vi "Umrechnung_Koordinaten.vi"(7 "Anderer Winkel":sgl, 8 "error in":errorcluster, 9 "Richtung":enum16{"Kamera nach Real", "Real nach Kamera"}(ring), 10 "Koordinaten in":cluster{"X":sgl, "Y":sgl}, 11 "Cluster in":T1={"Initialisierung"={"Online?"=FALSE, "Grundpfad"=path "", "Kamera Oben"="", "IP-Adresse Flüssiglinse"="", "Flüssiglinse"=refnum, "Kamera Unten"="", "IP-Adresse SPS"="", "SPS-Verbindung"={"TCP Connection Ref"=refnum, "IP address"="", "timeout ms"=5000, "Connected?"=FALSE, "PLC Type"=enum."S7 1200", "Rack S7 400"=0, "Slot S7 400"=0, "PDU Size"=0, "connection semaphore"=refnum}, "IP-Adresse Lichtgitter"="", "Lichtgitter"=refnum, "Skalierungsfaktor"=0.0, "Bilder Oben"=[], "Bild Unten"=refnum, "Bild Ausschnitt Unten"=refnum}, "Einstellungen"={"Gesamtablauf gestartet"=FALSE, "i. O. Bilder speichern"=FALSE, "Bildspeicherung Offline"=FALSE, "Ausgewähltes Offline-Datum"="", "Ausgewähltes Offline-Teil"="", "Speicherpfad Bilder"=path ""}, "Artikeldaten"={"Artikelnummer"="", "Fertigungsauftrag"="", "Muster ISO"=refnum, "Belichtungszeit Referenzmarken"=0.0, "Fokus Referenzmarken"=0.0, "Belichtungszeit ISO"=0.0, "Fokus ISO"=0.0, "Belichtungszeit Unten"=0.0, "Kontaktanzahl"=0, "Aktueller Kontakt"=0, "Kontaktposition"={"x"=0.0, "y"=0.0}, "Winkel ISO"=0.0, "ISO-Muster nicht vorhanden"=FALSE}, "Werte Kamera Oben"={"Koordinatensystem"={"Punkt x-Achse"={"X"=0.0, "Y"=0.0}, "Ursprung"={"X"=0.0, "Y"=0.0}, "Punkt y-Achse"={"X"=0.0, "Y"=0.0}}, "Position Kontakt"={"x"=0.0, "y"=0.0}, "Winkel Kontakt"=0.0}, "Werte Kamera Unten"={"Prüfung Unten n. i. O."=FALSE}, "Werte Lichtgitter"={"Messwerte Referenzmarken"=[], "Mittelpunkt Referenzmarken"={"x"=0.0, "y"=0.0}, "Messwerte Kontakt"=[], "Offset"={"x"=0.0, "y"=0.0}}, "Rückmeldungen"={"Koordinaten ermittelt"=FALSE, "Vermessung Lichtgitter fertig"=FALSE, "Nachkontrolle Kamera Unten fertig"=FALSE}, "Fehler"={"Referenzen nicht gefunden"=FALSE, "Kontakt nicht gefunden"=FALSE, "Referenzen nicht in Lichtgitter"=FALSE, "Kontakt zu groß"=FALSE, "Kontakt zu klein"=FALSE}, "Statistik"={"Statistiken"=[]}, "Timer"={"Timer Start Position"=0, "Timer Start Lichtgitter"=0, "Timer Start Kamera Unten"=0}}) -> (0 "error out":errorcluster, 2 "Koordinaten out":cluster{"X":sgl, "Y":sgl}, 3 "Cluster out":T1={"Initialisierung"={"Online?"=FALSE, "Grundpfad"=path "", "Kamera Oben"="", "IP-Adresse Flüssiglinse"="", "Flüssiglinse"=refnum, "Kamera Unten"="", "IP-Adresse SPS"="", "SPS-Verbindung"={"TCP Connection Ref"=refnum, "IP address"="", "timeout ms"=5000, "Connected?"=FALSE, "PLC Type"=enum."S7 1200", "Rack S7 400"=0, "Slot S7 400"=0, "PDU Size"=0, "connection semaphore"=refnum}, "IP-Adresse Lichtgitter"="", "Lichtgitter"=refnum, "Skalierungsfaktor"=0.0, "Bilder Oben"=[], "Bild Unten"=refnum, "Bild Ausschnitt Unten"=refnum}, "Einstellungen"={"Gesamtablauf gestartet"=FALSE, "i. O. Bilder speichern"=FALSE, "Bildspeicherung Offline"=FALSE, "Ausgewähltes Offline-Datum"="", "Ausgewähltes Offline-Teil"="", "Speicherpfad Bilder"=path ""}, "Artikeldaten"={"Artikelnummer"="", "Fertigungsauftrag"="", "Muster ISO"=refnum, "Belichtungszeit Referenzmarken"=0.0, "Fokus Referenzmarken"=0.0, "Belichtungszeit ISO"=0.0, "Fokus ISO"=0.0, "Belichtungszeit Unten"=0.0, "Kontaktanzahl"=0, "Aktueller Kontakt"=0, "Kontaktposition"={"x"=0.0, "y"=0.0}, "Winkel ISO"=0.0, "ISO-Muster nicht vorhanden"=FALSE}, "Werte Kamera Oben"={"Koordinatensystem"={"Punkt x-Achse"={"X"=0.0, "Y"=0.0}, "Ursprung"={"X"=0.0, "Y"=0.0}, "Punkt y-Achse"={"X"=0.0, "Y"=0.0}}, "Position Kontakt"={"x"=0.0, "y"=0.0}, "Winkel Kontakt"=0.0}, "Werte Kamera Unten"={"Prüfung Unten n. i. O."=FALSE}, "Werte Lichtgitter"={"Messwerte Referenzmarken"=[], "Mittelpunkt Referenzmarken"={"x"=0.0, "y"=0.0}, "Messwerte Kontakt"=[], "Offset"={"x"=0.0, "y"=0.0}}, "Rückmeldungen"={"Koordinaten ermittelt"=FALSE, "Vermessung Lichtgitter fertig"=FALSE, "Nachkontrolle Kamera Unten fertig"=FALSE}, "Fehler"={"Referenzen nicht gefunden"=FALSE, "Kontakt nicht gefunden"=FALSE, "Referenzen nicht in Lichtgitter"=FALSE, "Kontakt zu groß"=FALSE, "Kontakt zu klein"=FALSE}, "Statistik"={"Statistiken"=[]}, "Timer"={"Timer Start Position"=0, "Timer Start Lichtgitter"=0, "Timer Start Kamera Unten"=0}})   [LabVIEW 2024]
uses:
  Cluster.ctl
  Kontaktmontagemodul.exe/1abvi3w/vi.lib/userDefined/High Color/IMAQdx.ctl
  Kontaktmontagemodul.exe/1abvi3w/vi.lib/DATA AHEAD/SP7/typedefs/S7 Connection.ctl
  Kontaktmontagemodul.exe/1abvi3w/vi.lib/DATA AHEAD/SP7/typedefs/PLC Type.ctl
  Kontaktmontagemodul.exe/1abvi3w/vi.lib/vision/Image Controls.llb/IMAQ Image.ctl
  Koordinatensystem.ctl
  Statistik.ctl
  Kontaktmontagemodul.exe/1abvi3w/vi.lib/vision/NI_Vision_Development_Module.lvlib
  Kontaktmontagemodul.exe/1abvi3w/vi.lib/Analysis/Matrix/NI_Matrix.lvlib
  Kontaktmontagemodul.exe/1abvi3w/vi.lib/DATA AHEAD/SP7/SP7.lvlib
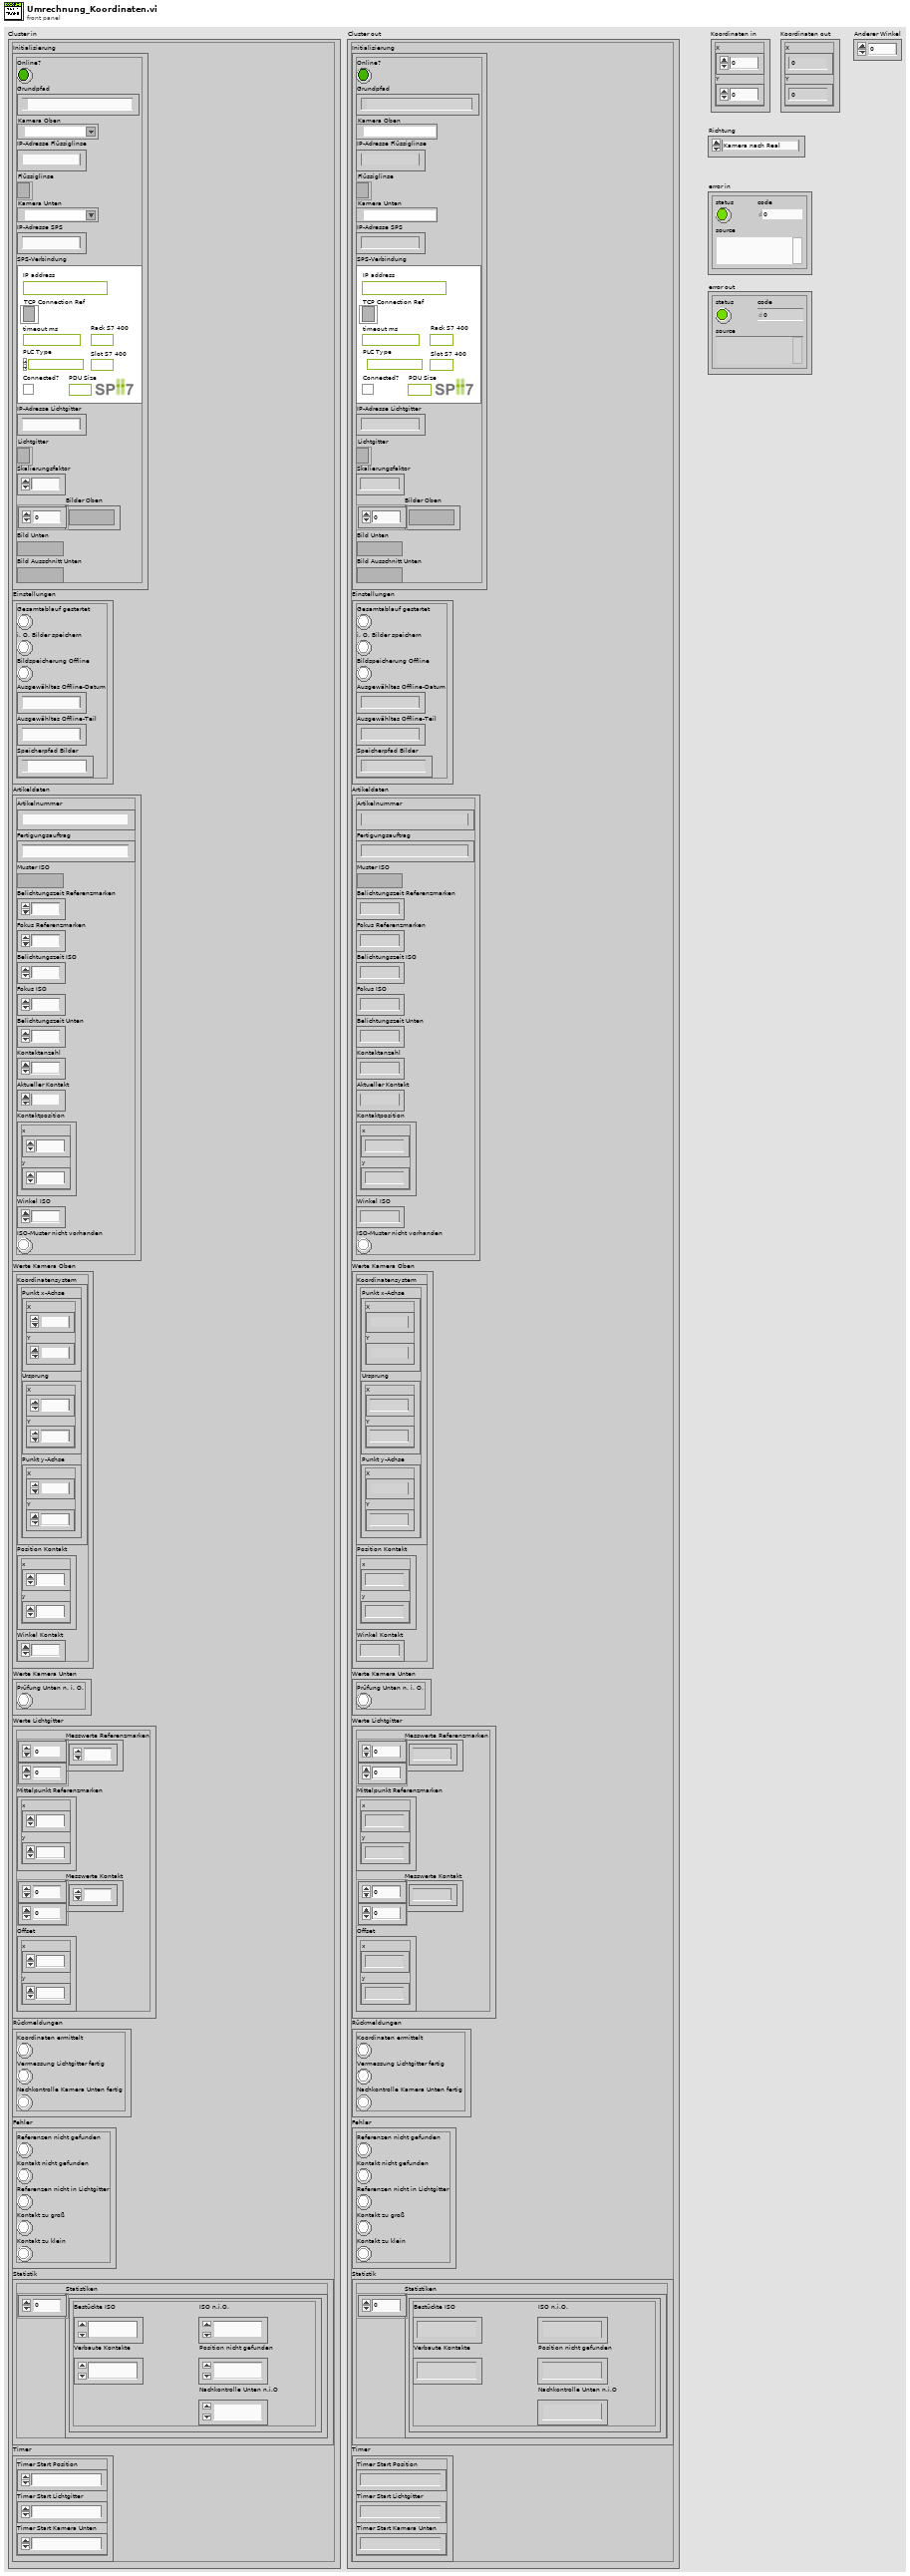
[diagram p1: front panel]
types:
  T1 = typedef "Cluster.ctl" = cluster{"Initialisierung":cluster{"Online?":bool, "Grundpfad":path, "Kamera Oben":T2, "IP-Adresse Flüssiglinse":string, "Flüssiglinse":refnum<k5>, "Kamera Unten":T2, "IP-Adresse SPS":string, "SPS-Verbindung":T3, "IP-Adresse Lichtgitter":string, "Lichtgitter":refnum<k5>, "Skalierungsfaktor":dbl, "Bilder Oben":T6[], "Bild Unten":T6, "Bild Ausschnitt Unten":T6}, "Einstellungen":cluster{"Gesamtablauf gestartet":bool, "i. O. Bilder speichern":bool, "Bildspeicherung Offline":bool, "Ausgewähltes Offline-Datum":string, "Ausgewähltes Offline-Teil":string, "Speicherpfad Bilder":path}, "Artikeldaten":cluster{"Artikelnummer":string, "Fertigungsauftrag":string, "Muster ISO":T6, "Belichtungszeit Referenzmarken":dbl, "Fokus Referenzmarken":dbl, "Belichtungszeit ISO":dbl, "Fokus ISO":dbl, "Belichtungszeit Unten":dbl, "Kontaktanzahl":u32, "Aktueller Kontakt":i16, "Kontaktposition":cluster{"x":sgl, "y":sgl}, "Winkel ISO":sgl, "ISO-Muster nicht vorhanden":bool}, "Werte Kamera Oben":cluster{"Koordinatensystem":T7, "Position Kontakt":cluster{"x":dbl, "y":dbl}, "Winkel Kontakt":dbl}, "Werte Kamera Unten":cluster{"Prüfung Unten n. i. O.":bool}, "Werte Lichtgitter":cluster{"Messwerte Referenzmarken":dbl[][], "Mittelpunkt Referenzmarken":cluster{"x":dbl, "y":dbl}, "Messwerte Kontakt":dbl[][], "Offset":cluster{"x":dbl, "y":dbl}}, "Rückmeldungen":cluster{"Koordinaten ermittelt":bool, "Vermessung Lichtgitter fertig":bool, "Nachkontrolle Kamera Unten fertig":bool}, "Fehler":cluster{"Referenzen nicht gefunden":bool, "Kontakt nicht gefunden":bool, "Referenzen nicht in Lichtgitter":bool, "Kontakt zu groß":bool, "Kontakt zu klein":bool}, "Statistik":cluster{"Statistiken":T8[]}, "Timer":cluster{"Timer Start Position":u32, "Timer Start Lichtgitter":u32, "Timer Start Kamera Unten":u32}}
  T2 = typedef "IMAQdx.ctl" = refnum<k21>
  T3 = typedef "SP7.lvlib/S7 Connection.ctl" = cluster{"TCP Connection Ref":refnum<k5>, "IP address":string, "timeout ms":i32, "Connected?":bool, "PLC Type":T4, "Rack S7 400":u8, "Slot S7 400":u8, "PDU Size":u16, "connection semaphore":T5}
  T4 = typedef "SP7.lvlib/PLC Type.ctl" = enum16{"S7 200", "S7 300/400", "S7 1200", "S7 1500", "LOGO!8"}
  T5 = typedef "Semaphore RefNum" = refnum<k1>
  T6 = typedef "IMAQ Image.ctl" = refnum<image>
  T7 = typedef "Koordinatensystem.ctl" = cluster{"Punkt x-Achse":cluster{"X":sgl, "Y":sgl}, "Ursprung":cluster{"X":sgl, "Y":sgl}, "Punkt y-Achse":cluster{"X":sgl, "Y":sgl}}
  T8 = typedef "Statistik.ctl" = cluster{"Bestückte ISO":u32, "Verbaute Kontakte":u32, "ISO n.i.O.":u32, "Nachkontrolle Unten n.i.O":u32, "Position nicht gefunden":u32}
  T9 = typedef "NI_Matrix.lvlib/RealMatrix.ctl" = dbl[][]
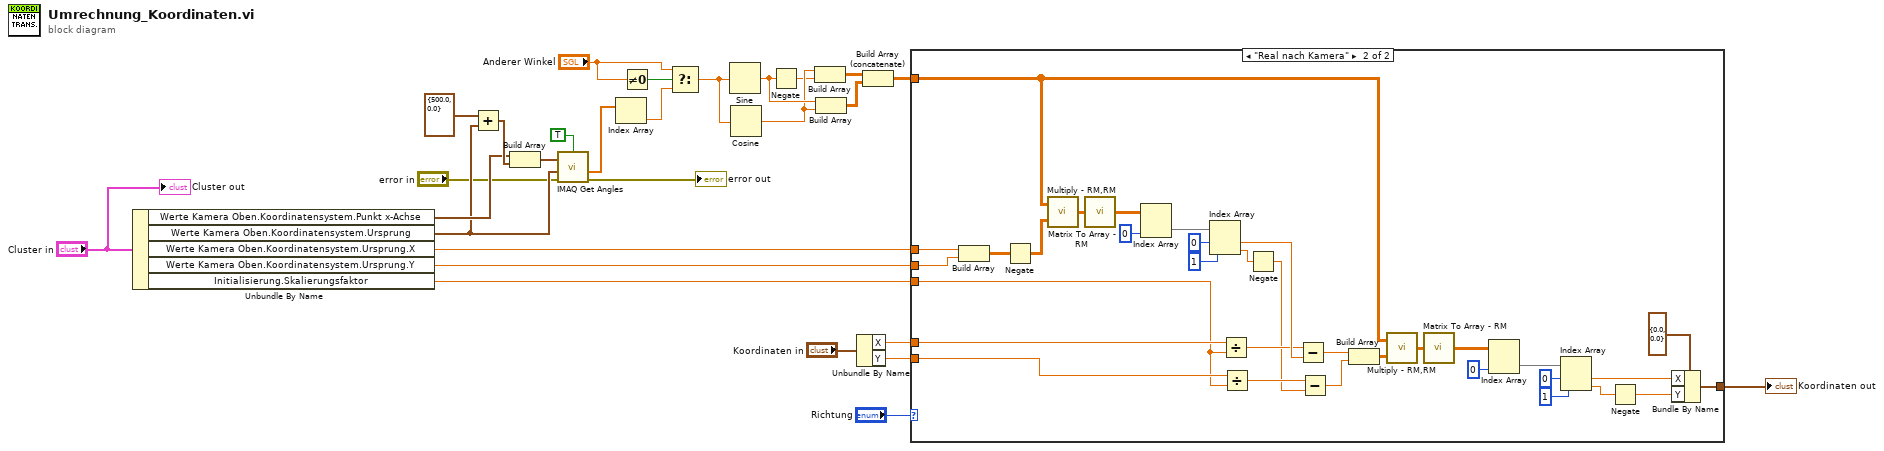
[diagram p0: block diagram]
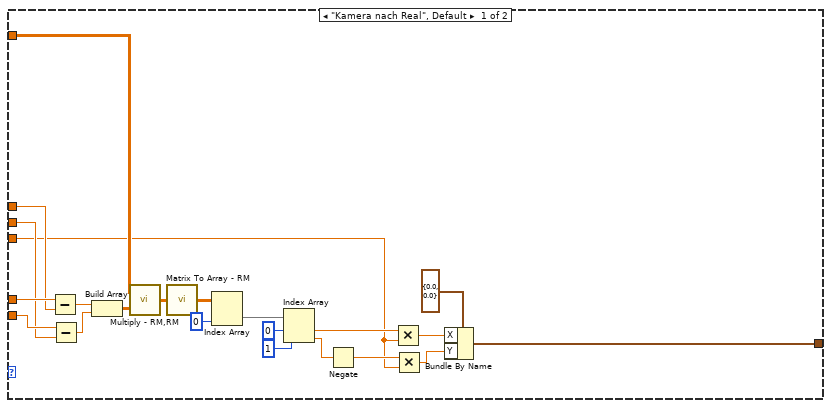
[diagram p2: hidden frame]
diagram:
  n1 = Unbundle By Name("Cluster in") -> ("Werte Kamera Oben.Koordinatensystem.Punkt x-Achse"=w9:cluster{"X":sgl, "Y":sgl}, "Werte Kamera Oben.Koordinatensystem.Ursprung"=w8:cluster{"X":sgl, "Y":sgl}, "Werte Kamera Oben.Koordinatensystem.Ursprung.X"=w27:sgl, "Werte Kamera Oben.Koordinatensystem.Ursprung.Y"=w21:sgl, "Initialisierung.Skalierungsfaktor"=w22:dbl)
  n2 = Add(x=cluster{"X":sgl, "Y":sgl} {"X"=500.0, "Y"=0.0} ("y"), y=w8) -> (x+y=w13:cluster{"X":sgl, "Y":sgl})
  n3 = Build Array(w9, w13) -> (w12:cluster{"X":sgl, "Y":sgl}[])
  n4 = call "IMAQ Get Angles"("error in (no error)"="error in", "Vertex"=w8, "Points"=w12, "Use Vertex (No)"=TRUE) -> ("error out"=→"error out":errorcluster, "Angles (rad)"=w14:sgl[])  [unwired: 1 in, 1 out]
  n5 = Index Array(array=w14) -> (element=w2:sgl)  [unwired: 1 in]
  n6 = Not Equal To 0?(x="Anderer Winkel") -> (x != 0?=w4:bool)
  n7 = Select(t="Anderer Winkel", s=w4, f=w2) -> (s? t:f=w1:sgl)
  n8 = Sine(x=w1) -> (sin(x)=w19:sgl)
  n9 = Cosine(x=w1) -> (cos(x)=w18:sgl)
  n10 = Negate(x=w19) -> (-x=w17:sgl)
  n11 = Build Array(w18, w17) -> (w15:T9)
  n12 = Build Array(w19, w18) -> (w16:T9)
  n13 = Unbundle By Name("Koordinaten in") -> ("X"=w24:sgl, "Y"=w23:sgl)
  n14 = Build Array (concatenate)(w15, w16) -> (w5:T9)
  n15 = case shown="\"Real nach Kamera\"" "Richtung" {
    tunnel: w27 -> [w41 w68]
    tunnel: [w31 w64] -> w25
    tunnel: w24 -> [w48 w63]
    tunnel: w23 -> [w40 w62]
    tunnel: w22 -> [w29 w51]
    tunnel: w21 -> [w39 w57]
    tunnel: w5 -> [w30 w52]
    frame "Kamera nach Real", Default {
      n16 = Subtract(x=w48, y=w41) -> (x-y=w50:sgl)
      n17 = Subtract(x=w40, y=w39) -> (x-y=w49:sgl)
      n18 = Build Array(w50, w49) -> (w38:T9)
      n19 = call "Multiply - RM,RM.vi"("Real Matrix B"=w38, "Real Matrix A"=w30) -> ("A * B"=w44:T9)
      n20 = call "Matrix To Array - RM.vi"("Real Matrix"=w44) -> ("Real 2D Array"=w45:dbl[][])
      n21 = Index Array(array=w45, index (col)=0 ("disabled index (col)")) -> (element=w42:dbl[])  [unwired: 1 in]
      n22 = Index Array(array=w42, index #1=0 ("index"), index #2=1 ("index")) -> (element #1=w35:dbl, element #2=w36:dbl)
      n23 = Negate(x=w36) -> (-x=w33:dbl)
      n24 = Multiply(x=w35, y=w29) -> (x*y=w34:dbl)
      n25 = Multiply(x=w33, y=w29) -> (x*y=w32:dbl)
      n26 = Bundle By Name(cluster=cluster{"X":sgl, "Y":sgl} {"X"=0.0, "Y"=0.0} ("Koordinaten out"), "X"=w34, "Y"=w32) -> (w31:cluster{"X":sgl, "Y":sgl})
    }
    frame "Real nach Kamera" {
      n27 = Build Array(w68, w57) -> (w56:T9)
      n28 = Negate(x=w56) -> (-x=w55:T9)
      n29 = call "Multiply - RM,RM.vi"("Real Matrix B"=w55, "Real Matrix A"=w52) -> ("A * B"=w76:T9)
      n30 = call "Matrix To Array - RM.vi"("Real Matrix"=w76) -> ("Real 2D Array"=w75:dbl[][])
      n31 = Index Array(array=w75, index (col)=0 ("disabled index (col)")) -> (element=w69:dbl[])  [unwired: 1 in]
      n32 = Index Array(array=w69, index #1=0 ("index"), index #2=1 ("index")) -> (element #1=w72:dbl, element #2=w54:dbl)
      n33 = Divide(x=w63, y=w51) -> (x/y=w61:dbl)
      n34 = Divide(x=w62, y=w51) -> (x/y=w60:dbl)
      n35 = Negate(x=w54) -> (-x=w53:dbl)
      n36 = Subtract(x=w61, y=w72) -> (x-y=w71:dbl)
      n37 = Subtract(x=w60, y=w53) -> (x-y=w70:dbl)
      n38 = Build Array(w71, w70) -> (w78:T9)
      n39 = call "Multiply - RM,RM.vi"("Real Matrix B"=w78, "Real Matrix A"=w52) -> ("A * B"=w80:T9)
      n40 = call "Matrix To Array - RM.vi"("Real Matrix"=w80) -> ("Real 2D Array"=w81:dbl[][])
      n41 = Index Array(array=w81, index (col)=0 ("disabled index (col)")) -> (element=w67:dbl[])  [unwired: 1 in]
      n42 = Index Array(array=w67, index #1=0 ("index"), index #2=1 ("index")) -> (element #1=w58:dbl, element #2=w66:dbl)
      n43 = Negate(x=w66) -> (-x=w59:dbl)
      n44 = Bundle By Name(cluster=cluster{"X":sgl, "Y":sgl} {"X"=0.0, "Y"=0.0} ("Koordinaten out"), "X"=w58, "Y"=w59) -> (w64:cluster{"X":sgl, "Y":sgl})
    }
  }
  "Koordinaten out" <- w25
  "Cluster out" <- "Cluster in"
